vi "Create Stoopid Segment Velocities.vi"(9 "Conditions":T1, 10 "Velocities":dbl[](array[numeric]), 11 "Limits":T2={"Velocity (fps)"=6.0, "Accel (fps^2)"=15.0, "Jerk (fps^3)"=150.0, "StoopidFast (fps)"=6.0} {"StoopidFast (fps)" min=0.0; "Jerk (fps^3)" min=0.0 step=1.0; "Accel (fps^2)" min=0.0; "Velocity (fps)" min=0.0}) -> (3 "Velocities":dbl[](array[numeric]))   [LabVIEW 2019]
uses:
  Types/Limits.ctl
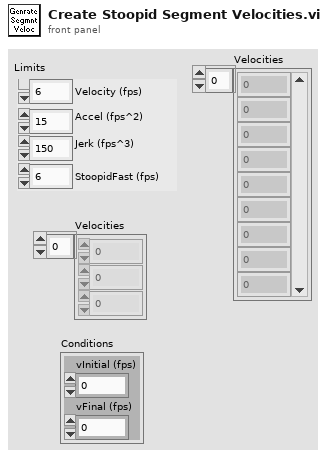
[diagram p1: front panel]
types:
  T1 = cluster{"vInitial (fps)":dbl, "vFinal (fps)":dbl}
  T2 = typedef "Limits.ctl" = cluster{"Velocity (fps)":dbl, "Accel (fps^2)":dbl, "Jerk (fps^3)":dbl, "StoopidFast (fps)":dbl}
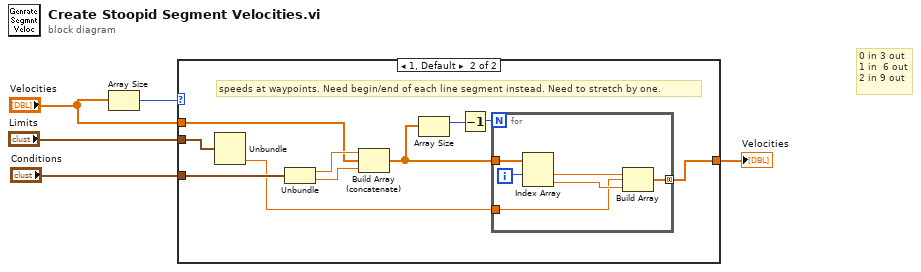
[diagram p0: block diagram]
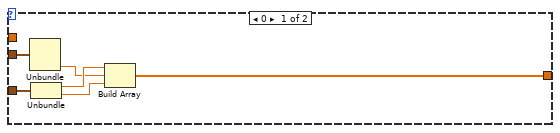
[diagram p2: hidden frame]
diagram:
  # "0 in 3 out\n1 in  6 out\n2 in 9 out"
  n1 = Array Size(array="Velocities") -> (size(s)=w1:i32)
  n2 = case shown="1, Default" w1 {
    tunnel: "Conditions" -> [w11 w19]
    tunnel: "Velocities" -> [_ w18]
    tunnel: "Limits" -> [w10 w13]
    tunnel: [w7 w14] -> w5
    frame 0 {
      n3 = Unbundle(w10) -> ("StoopidFast (fps)"=w6:dbl)  [unwired: 3 out]
      n4 = Unbundle(w11) -> ("vInitial (fps)"=w9:dbl, "vFinal (fps)"=w8:dbl)
      n5 = Build Array(w9, w6, w8) -> (w7:dbl[])
    }
    frame 1, Default {
      # "speeds at waypoints. Need begin/end of each line segment instead. Need to stretch by one."
      n6 = Unbundle(w13) -> ("StoopidFast (fps)"=w12:dbl)  [unwired: 3 out]
      n7 = Unbundle(w19) -> ("vInitial (fps)"=w21:dbl, "vFinal (fps)"=w20:dbl)
      n8 = Build Array (concatenate)(w21, w18, w20) -> (w15:dbl[])
      n9 = Array Size(array=w15) -> (size(s)=w16:i32)
      n10 = Decrement(x=w16) -> (x-1=w17:i32)
      n11 = for {
        N: w17 -> [_]
        tunnel: w15 -> [w27]
        tunnel: [w23] -> w14 mode=concatenating
        tunnel: w12 -> [w22]
        i -> [w26]
        n12 = Index Array(array=w27, index #1=w26) -> (element #1=w25:dbl, element #2=w24:dbl)  [unwired: 1 in]
        n13 = Build Array(w25, w22, w24) -> (w23:dbl[])
      }
    }
  }
  "Velocities" <- w5
